vi "Suppress Teardown Error.vi"(10 "Error in":errorcluster) -> (2 "Error out":errorcluster)   [LabVIEW 2020, in "jettl.lvlib" / "Actor.lvlib"]
uses:
  Actor.lvlib
  Error/Error.lvlib
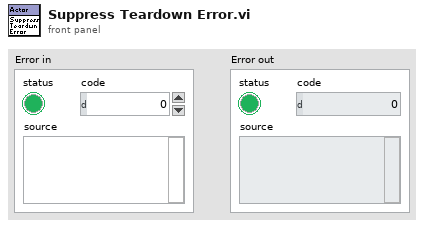
[diagram p1: front panel]
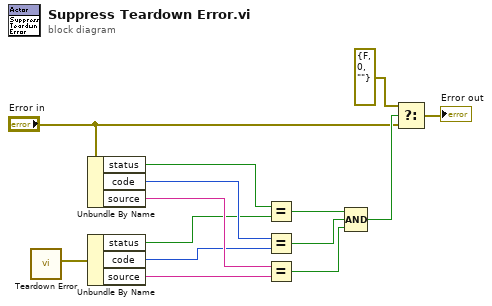
[diagram p0: block diagram]
diagram:
  n1 = call "Teardown Error.vi"() -> ("Error"=w14:errorcluster)  [unwired: 11 in]
  n2 = Unbundle By Name("Error in") -> ("status"=w13:bool, "code"=w12:i32, "source"=w11:string)
  n3 = Unbundle By Name(w14) -> ("status"=w10:bool, "code"=w9:i32, "source"=w8:string)
  n4 = Equal?(x=w13, y=w10) -> (x = y?=w7:bool)
  n5 = Equal?(x=w12, y=w9) -> (x = y?=w6:bool)
  n6 = Equal?(x=w11, y=w8) -> (x = y?=w5:bool)
  n7 = Compound Arithmetic op=AND(w7, w6, w5) -> (w4:bool)
  n8 = Select(t=errorcluster {"status"=FALSE, "code"=0, "source"=""}, s=w4, f="Error in") -> (s? t:f=→"Error out":errorcluster)
